vi "test Encapsulate.vi"(8 "error in (no error)":errorcluster, 11 "TestCase in":refnum<class "Lifecycle Tests.lvclass">) -> (0 "error out":errorcluster, 3 "TestCase out":refnum<class "Lifecycle Tests.lvclass">)   [LabVIEW 2020, in "Memory Manager Tests.lvlib" / "Lifecycle Tests.lvclass"]
uses:
  Lifecycle Tests.lvclass
  C:/Program Files/National Instruments/LabVIEW 2027/vi.lib/addons/_JKI Toolkits/VI Tester/TestCase.llb/TestCase.lvclass
  <vilib>/addons/_JKI Toolkits/VI Tester/TestCase.llb/TestCase.lvclass
  Classes/Pointer/Pointer.lvclass
  Classes/Pointer/Read I32.vi
  Classes/Pointer/Write 1D I32.vi
  Classes/Pointer/Write I32.vi
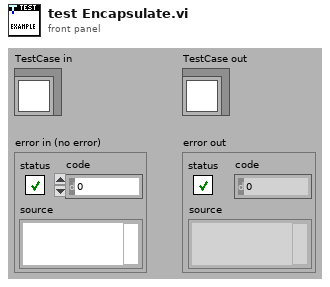
[diagram p1: front panel]
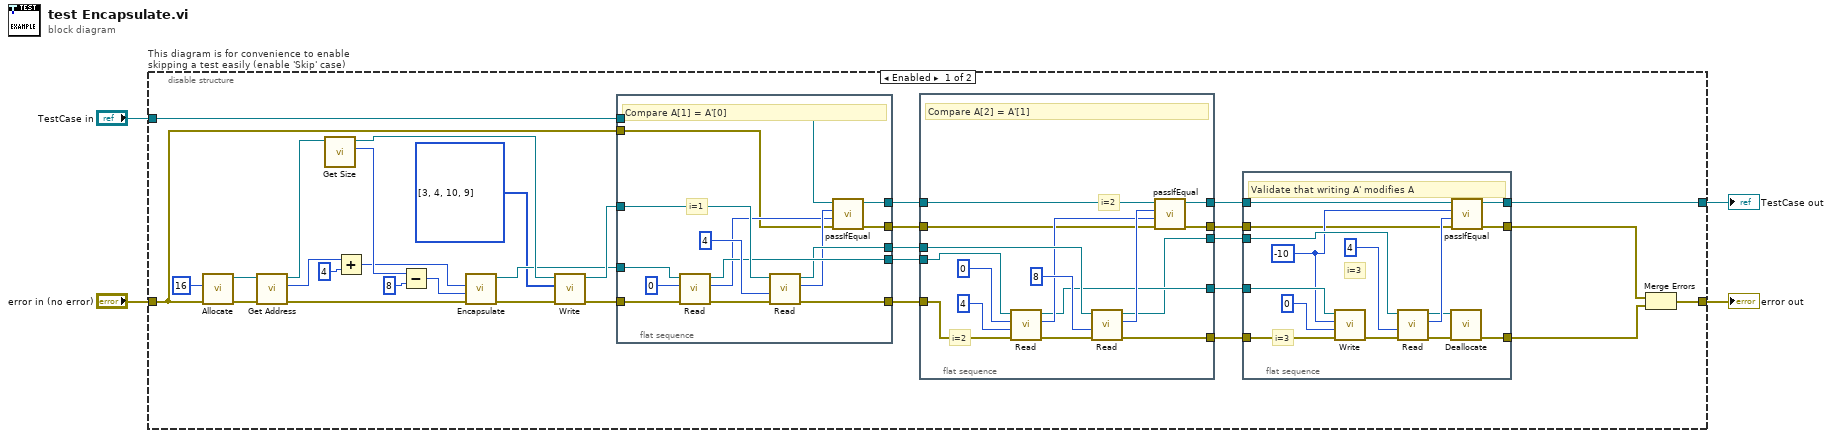
[diagram p0: block diagram]
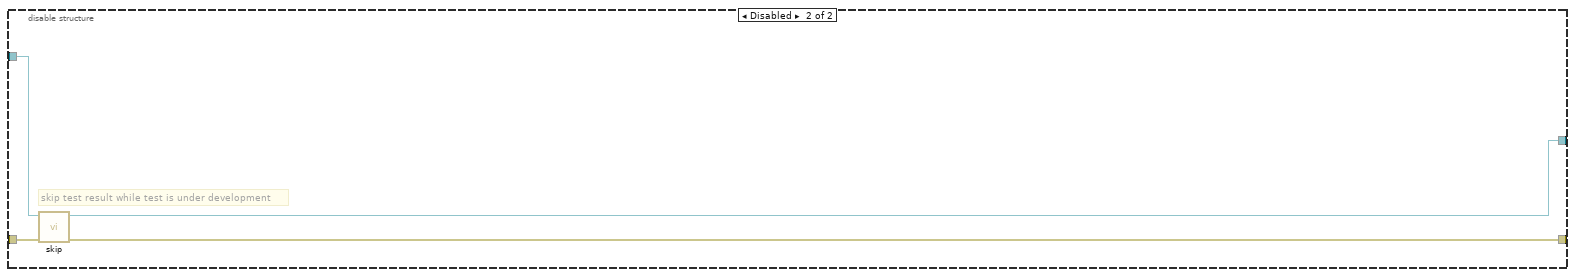
[diagram p2: hidden frame]
diagram:
  n1 = disable-structure "This diagram is for convenience to enable skipping a test easily (enable 'Skip' case)" shown="Enabled" {
    disable-tunnel: "TestCase in" -> [w12 w86]
    disable-tunnel: [w9 w84] -> w1
    disable-tunnel: [w22 w85] -> w3
    disable-tunnel: "error in (no error)" -> [w8 w83]
    frame Enabled {
      n2 = call "Allocate.vi"("error in (no error)"=w8, "size"=u64 16 ("count (1)")) -> ("error out"=w29:errorcluster, "Pointer out"=w6:refnum<class "Pointer.lvclass">)  [unwired: 8 in]
      n3 = call "Get Address.vi"("Pointer in"=w6) -> ("address"=w35:u64, "Pointer out"=w36:refnum<class "Pointer.lvclass">)  [unwired: 9 in]
      n4 = call "Get Size.vi"("Pointer in"=w36) -> ("size"=w33:u64, "Pointer out"=w28:refnum<class "Pointer.lvclass">)  [unwired: 9 in]
      n5 = Add(x=w35, y=u64 4) -> (x+y=w31:u64)
      n6 = Subtract(x=w33, y=u64 8) -> (x-y=w30:u64)
      n7 = call "Encapsulate.vi"("error in (no error)"=w29, "size"=w30, "address"=w31) -> ("error out"=w27:errorcluster, "Pointer"=w20:refnum<class "Pointer.lvclass">)  [unwired: 7 in]
      n8 = call-poly "Write.vi"("error in (no error)"=w27, "buffer in"=i32[] [3, 4, 10, 9] ("length (-1: rest)"), "Pointer in"=w28) -> ("error out"=w13:errorcluster, "Pointer out"=w26:refnum<class "Pointer.lvclass">)  [unwired: 5 in, 2 out]
      n9 = flat-sequence {
        tunnel: w26 -> [w82]
        tunnel: [w79] -> w25
        tunnel: [w78] -> w24
        tunnel: w20 -> [w75]
        tunnel: [w73] -> w19
        tunnel: [w72] -> w14
        tunnel: w13 -> [w71]
        tunnel: w12 -> [w70]
        tunnel: [w69] -> w11
        tunnel: w8 -> [w68]
        frame #0 {
          # "i=1"
          # "Compare A[1] = A'[0]"
          n10 = call-poly "Read.vi"("error in (no error)"=w71, "value in"=0 ("length (-1: rest)"), "Pointer in"=w75) -> ("error out"=w74:errorcluster, "value out"=w76:i32, "Pointer out"=w79:refnum<class "Pointer.lvclass">)  [unwired: 5 in, 1 out]
          n11 = call-poly "Read.vi"("error in (no error)"=w74, "offset (0)"=u64 4, "Pointer in"=w82) -> ("error out"=w72:errorcluster, "value out"=w77:i32, "Pointer out"=w78:refnum<class "Pointer.lvclass">)  [unwired: 5 in, 1 out]
          n12 = call-dynamic "passIfEqual.vi"("error in (no error)"=w68, "y"=w76, "x"=w77, "TestCase in"=w70) -> ("error out"=w73:errorcluster, "TestCase out"=w69:refnum<class "Lifecycle Tests.lvclass">)  [unwired: 6 in]
        }
      }
      n13 = flat-sequence {
        tunnel: w25 -> [w52]
        tunnel: w24 -> [w49]
        tunnel: [w45] -> w23
        tunnel: w19 -> [w43]
        tunnel: [w42] -> w18
        tunnel: [w41] -> w15
        tunnel: w14 -> [w40]
        tunnel: w11 -> [w39]
        tunnel: [w38] -> w10
        tunnel: [w37] -> w7
        frame #0 {
          # "i=2"
          # "i=2"
          # "Compare A[2] = A'[1]"
          n14 = call-poly "Read.vi"("error in (no error)"=w40, "offset (0)"=u64 4, "value in"=0 ("length (-1: rest)"), "Pointer in"=w52) -> ("error out"=w44:errorcluster, "value out"=w46:i32, "Pointer out"=w45:refnum<class "Pointer.lvclass">)  [unwired: 4 in, 1 out]
          n15 = call-poly "Read.vi"("error in (no error)"=w44, "offset (0)"=u64 8, "Pointer in"=w49) -> ("error out"=w41:errorcluster, "value out"=w47:i32, "Pointer out"=w37:refnum<class "Pointer.lvclass">)  [unwired: 5 in, 1 out]
          n16 = call-dynamic "passIfEqual.vi"("error in (no error)"=w43, "y"=w46, "x"=w47, "TestCase in"=w39) -> ("error out"=w42:errorcluster, "TestCase out"=w38:refnum<class "Lifecycle Tests.lvclass">)  [unwired: 6 in]
        }
      }
      n17 = flat-sequence {
        tunnel: w23 -> [w67]
        tunnel: w7 -> [w66]
        tunnel: w18 -> [w61]
        tunnel: [w60] -> w17
        tunnel: [w54] -> w16
        tunnel: w15 -> [w58]
        tunnel: w10 -> [w57]
        tunnel: [w56] -> w9
        frame #0 {
          w65 = -10 ("length (-1: rest)")
          # "i=3"
          # "i=3"
          # "Validate that writing A' modifies A"
          n18 = call-poly "Write.vi"("error in (no error)"=w58, "offset (0)"=u64 0, "value"=w65, "Pointer in"=w67) -> ("error out"=w62:errorcluster)  [unwired: 4 in, 3 out]
          n19 = call-poly "Read.vi"("error in (no error)"=w62, "offset (0)"=u64 4, "Pointer in"=w66) -> ("error out"=w59:errorcluster, "value out"=w63:i32, "Pointer out"=w53:refnum<class "Pointer.lvclass">)  [unwired: 5 in, 1 out]
          n20 = call "Deallocate.vi"("error in (no error)"=w59, "Pointer"=w53) -> ("error out"=w54:errorcluster)  [unwired: 8 in, 1 out]
          n21 = call-dynamic "passIfEqual.vi"("error in (no error)"=w61, "y"=w63, "x"=w65, "TestCase in"=w57) -> ("error out"=w60:errorcluster, "TestCase out"=w56:refnum<class "Lifecycle Tests.lvclass">)  [unwired: 6 in]
        }
      }
      n22 = Merge Errors(w17, w16) -> (w22:errorcluster)
    }
    frame Disabled {
      # "skip test result while test is under development"
      n23 = call <vilib>:"skip.vi"("error in (no error)"=w83, "TestCase in"=w86) -> ("error out"=w85:errorcluster, "TestCase out"=w84:refnum<class "Lifecycle Tests.lvclass">)  [unwired: 8 in]
    }
  }
  "error out" <- w3
  "TestCase out" <- w1
